vi "MEDIDOR 2.vi"() -> (0 "CORRENTE FASE A":dynamicdata(graph) caption="Waveform Graph", 1 "CORRENTE FASE B":dynamicdata(graph) caption="Waveform Graph", 2 "TENSAO FASE A":dynamicdata(graph) caption="Waveform Graph", 3 "TENSAO FASE B":dynamicdata(graph) caption="Waveform Graph")   [LabVIEW 2020]
panel:
  out "timestamp 10":string[][](table)
  out "CORRENTE FASE C":dynamicdata(graph) caption="Waveform Graph"
  out "TENSAO FASE C":dynamicdata(graph) caption="Waveform Graph"
  out "timestamp 7":string[][](table)
  out "timestamp":string[][](table)
  out "Table":string[][](table)
  out "timestamp":dynamicdata(graph) caption="Waveform Graph"
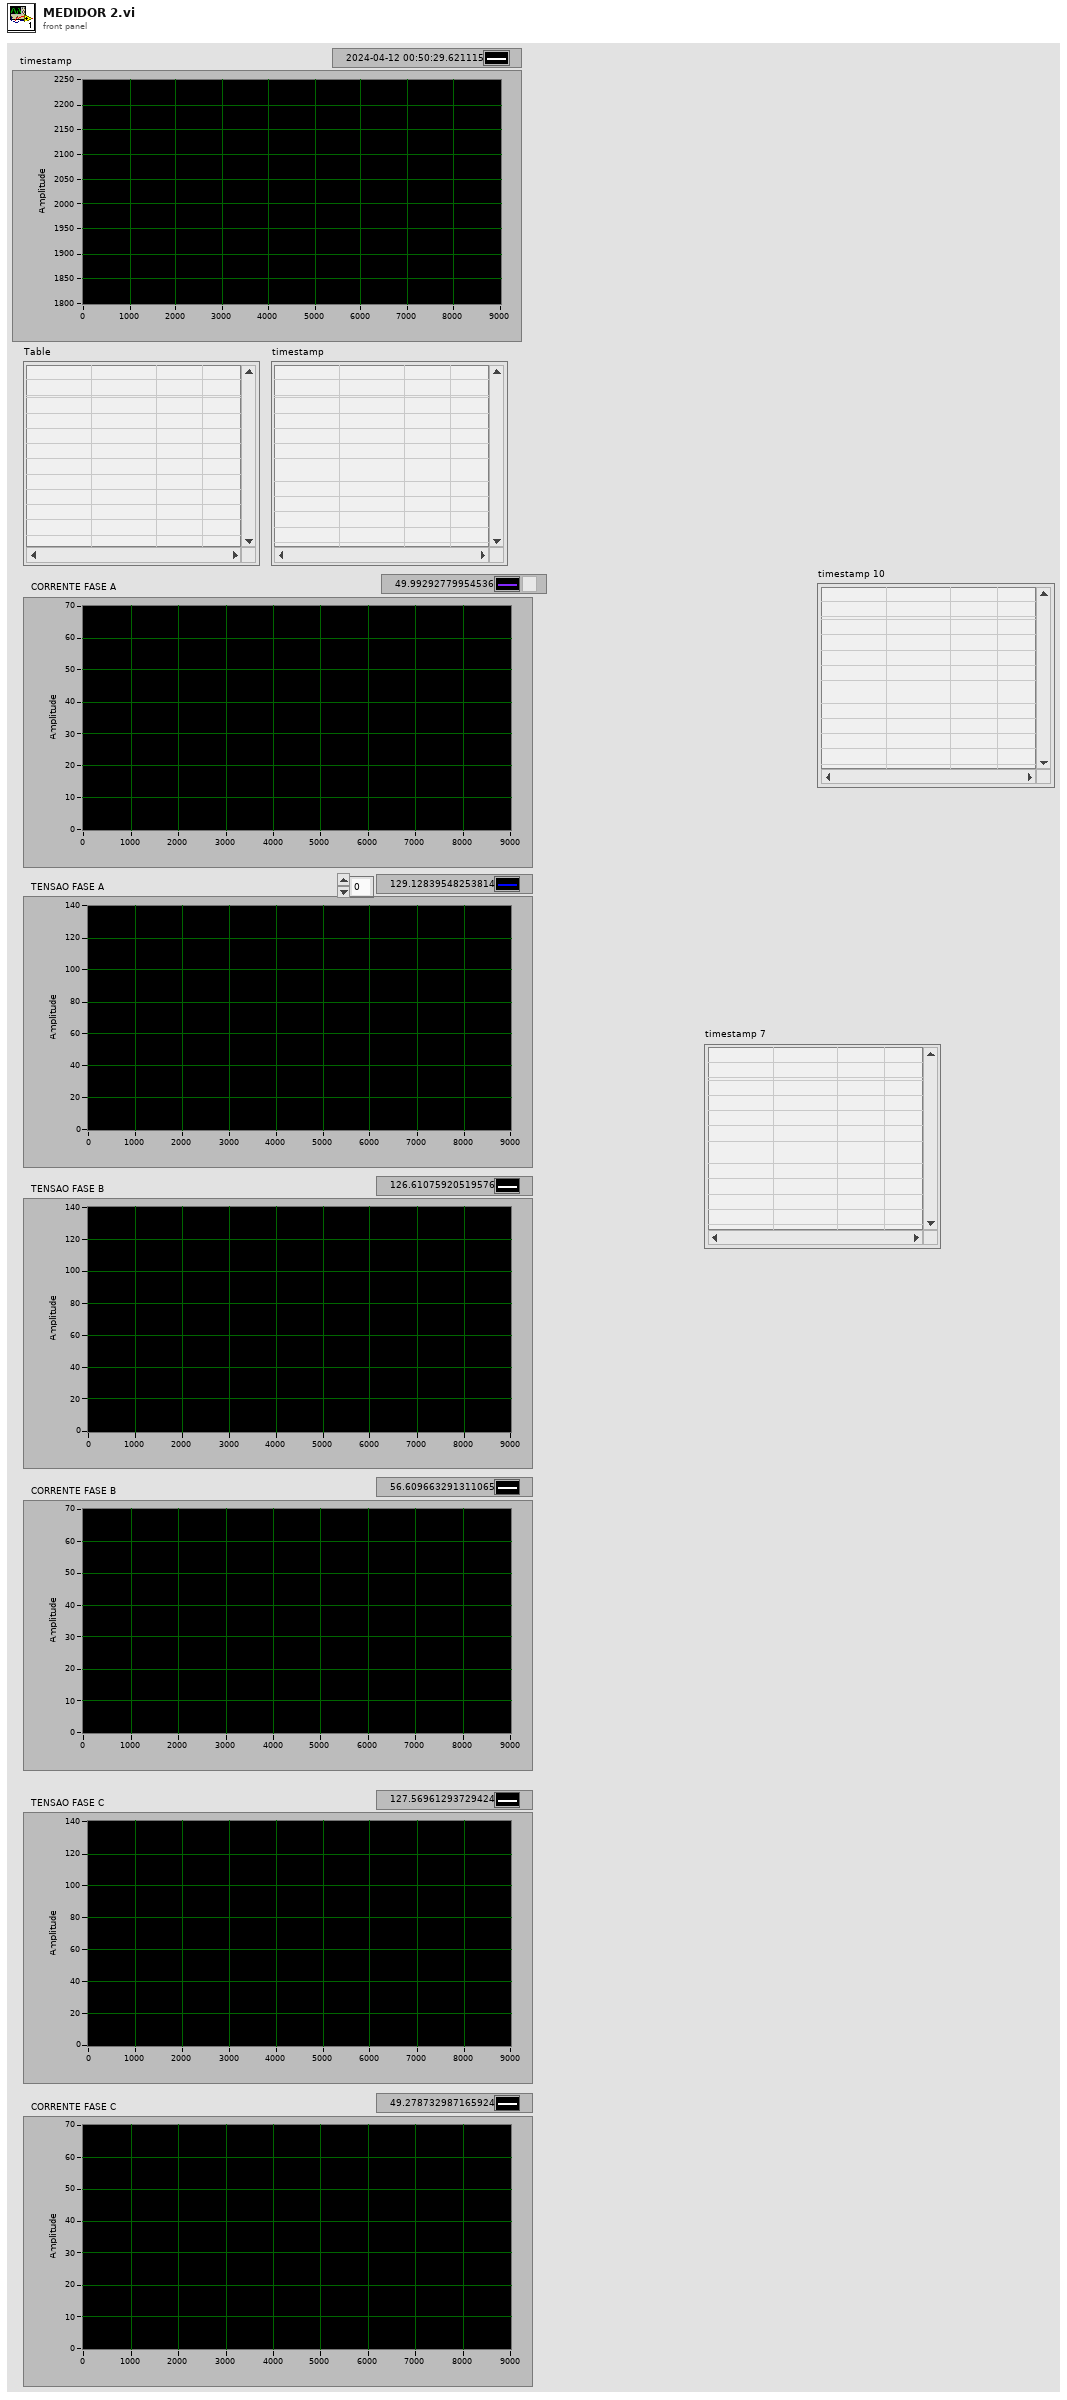
[diagram p1: front panel]
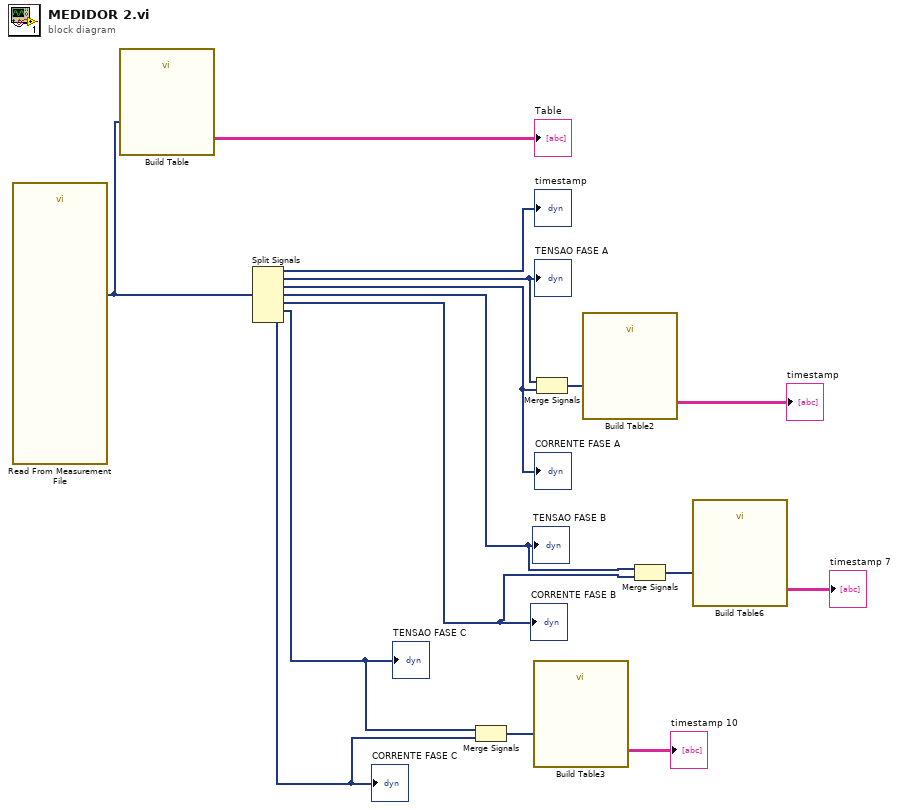
[diagram p0: block diagram]
diagram:
  n1 = call "Read From Measurement File"() -> ("Signals"=w14:dynamicdata)  [unwired: 6 in, 5 out]
  n2 = call "Build Table"("Signals"=w14) -> ("Table"=→"Table":string[][])  [unwired: 4 in, 6 out]
  n3 = Split Signals(w14) -> (→"timestamp":dynamicdata, w11:dynamicdata, w10:dynamicdata, w8:dynamicdata, w7:dynamicdata, w2:dynamicdata, w1:dynamicdata)  [unwired: 7 in]
  "CORRENTE FASE A" <- w10
  "TENSAO FASE A" <- w11
  "TENSAO FASE B" <- w8
  "CORRENTE FASE B" <- w7
  "TENSAO FASE C" <- w2
  "CORRENTE FASE C" <- w1
  n4 = Merge Signals(w2, w1) -> (w4:dynamicdata)
  n5 = call "Build Table3"("Signals"=w4) -> ("Table"=→"timestamp 10":string[][])  [unwired: 4 in, 6 out]
  n6 = Merge Signals(w11, w10) -> (w9:dynamicdata)
  n7 = call "Build Table2"("Signals"=w9) -> ("Table"=→"timestamp":string[][])  [unwired: 4 in, 6 out]
  n8 = Merge Signals(w8, w7) -> (w6:dynamicdata)
  n9 = call "Build Table6"("Signals"=w6) -> ("Table"=→"timestamp 7":string[][])  [unwired: 4 in, 6 out]
